vi "Test Bus of Buses.vi"() -> ()   [LabVIEW 2021]
uses:
  Source/Omni-Bus/Omni_Bus.lvclass
  Source/Omni-Bus/Support/Broad Types.ctl
  Source/Local Bus/Local Bus.lvclass
  <vilib>/Utility/Data Type/Type Definitions/Data Type.ctl
  <vilib>/Utility/Data Type/NI_Data Type.lvlib
  Source/Aggregator Bus/Aggregator Bus.lvclass
  C:/Users/Tim/Documents/GitHub/Omni-Bus/Source/Omni-Bus/Bus Access/Bus_Access.lvclass
  C:/Program Files (x86)/National Instruments/LabVIEW 2021/vi.lib/TSA/Abstract Data Classes/Abs_Types/Type/Abs_Type.lvclass
  C:/Users/Tim/Documents/GitHub/Omni-Bus/Source/Local Bus/Local Bus.lvclass
  Source/Omni-Bus/Support/Read/Read Time.vi
  Source/Omni-Bus/Support/Read/Read String.vi
  Source/Omni-Bus/Support/Read/Read Boolean.vi
  Source/Omni-Bus/Support/Write/Write String.vi
  Source/Omni-Bus/Support/Write/Write Boolean.vi
  <vilib>/TSA/Abstract Data Classes/Abs_Types/Time/Abs_Time.lvclass
  C:/Program Files (x86)/National Instruments/LabVIEW 2021/vi.lib/TSA/Abstract Data Classes/Abs_Types/Numeric/Abs_Numeric.lvclass
  C:/Program Files (x86)/National Instruments/LabVIEW 2021/vi.lib/TSA/Abstract Data Classes/Abs_Types/Value/Abs_Value.lvclass
  C:/Program Files (x86)/National Instruments/LabVIEW 2021/vi.lib/TSA/Abstract Data Classes/Abs_Types/Time/Abs_Time.lvclass
  C:/Users/Tim/Documents/GitHub/Omni-Bus/Source/Omni-Bus/Omni_Bus.lvclass
  C:/Users/Tim/Documents/GitHub/Omni-Bus/Source/Aggregator Bus/Aggregator Bus.lvclass
panel:
  in  "A 3":bool
  in  "B 3":dbl
  in  "C 3":string
  out "A 2":bool
  out "B 2":dbl
  out "C 2":string
  out "Time Stamp":timestamp
  in  "C":string
  in  "B":dbl
  in  "A":bool
  out "C":string
  out "B":dbl
  out "A":bool
  out "error out 3":errorcluster
  out "error out 2":errorcluster
  in  "Numeric 2":dbl
  in  "Tag 2":string
  in  "stop":bool
  out "Numeric":dbl
  in  "Tag":string
  out "error out":errorcluster
  out "Tags":string[](array[string])
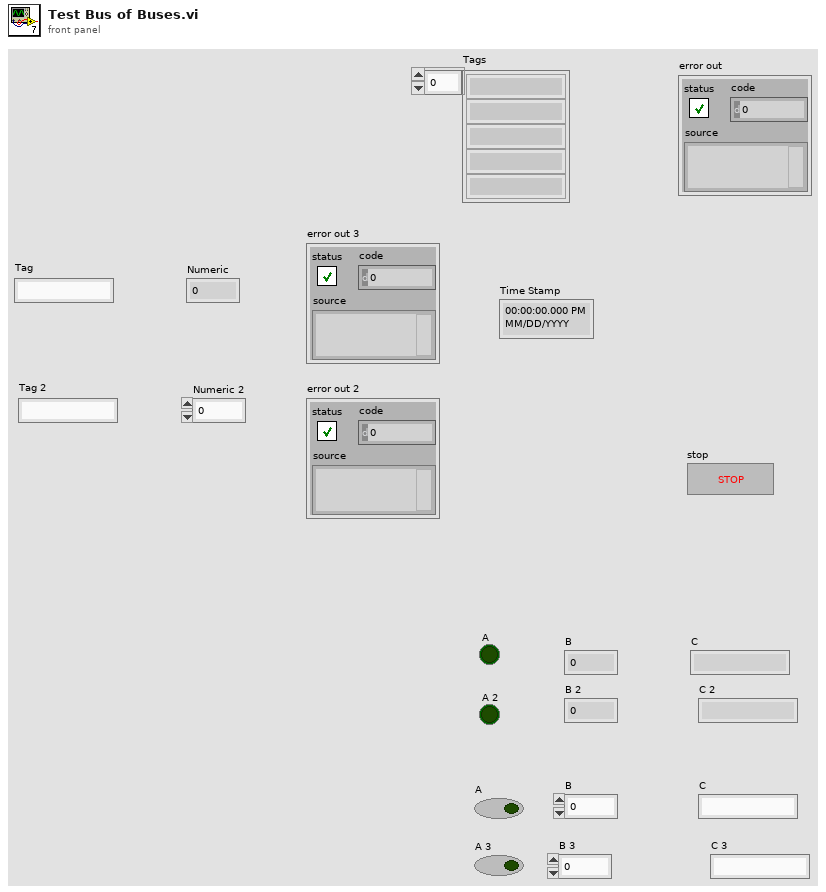
[diagram p1: front panel]
types:
  T1 = typedef "NI_Data Type.lvlib/Data Type.ctl" = enum8{"Invalid Type", "Void", "I8", "I16", "I32", "I64", "U8", "U16", "U32", "U64", "Single Float", "Double Float", "Extended Float", "Single Complex", "Double Complex", "Extended Complex", "Enum U8", "Enum U16", "Enum U32", "Enum U64", "Single Float With Unit", "Double Float With Unit", "Extended Float With Unit", "Single Complex with Unit", "Double Complex with Unit", "Extended Complex with Unit", "Boolean", "String", "Path", "Picture", "Tag", "Array", "Cluster", "Variant", "LV Variant", "Waveform", "Timestamp", "Digital Waveform", "Digital Data", "ExpressData", "Refnum", "External Data", "VI", "Poly VI", "LabVIEW Class Instance", "Fixed Point", "Set Collection", "Map Collection"}
  T2 = typedef "Omni_Bus.lvclass/Broad Types.ctl" = enum16{"All Tags", "NI Specific Type", "Boolean", "String", "Numeric", "Float", "Integer", "Collection", "All Value Types", "Non Value Types"}
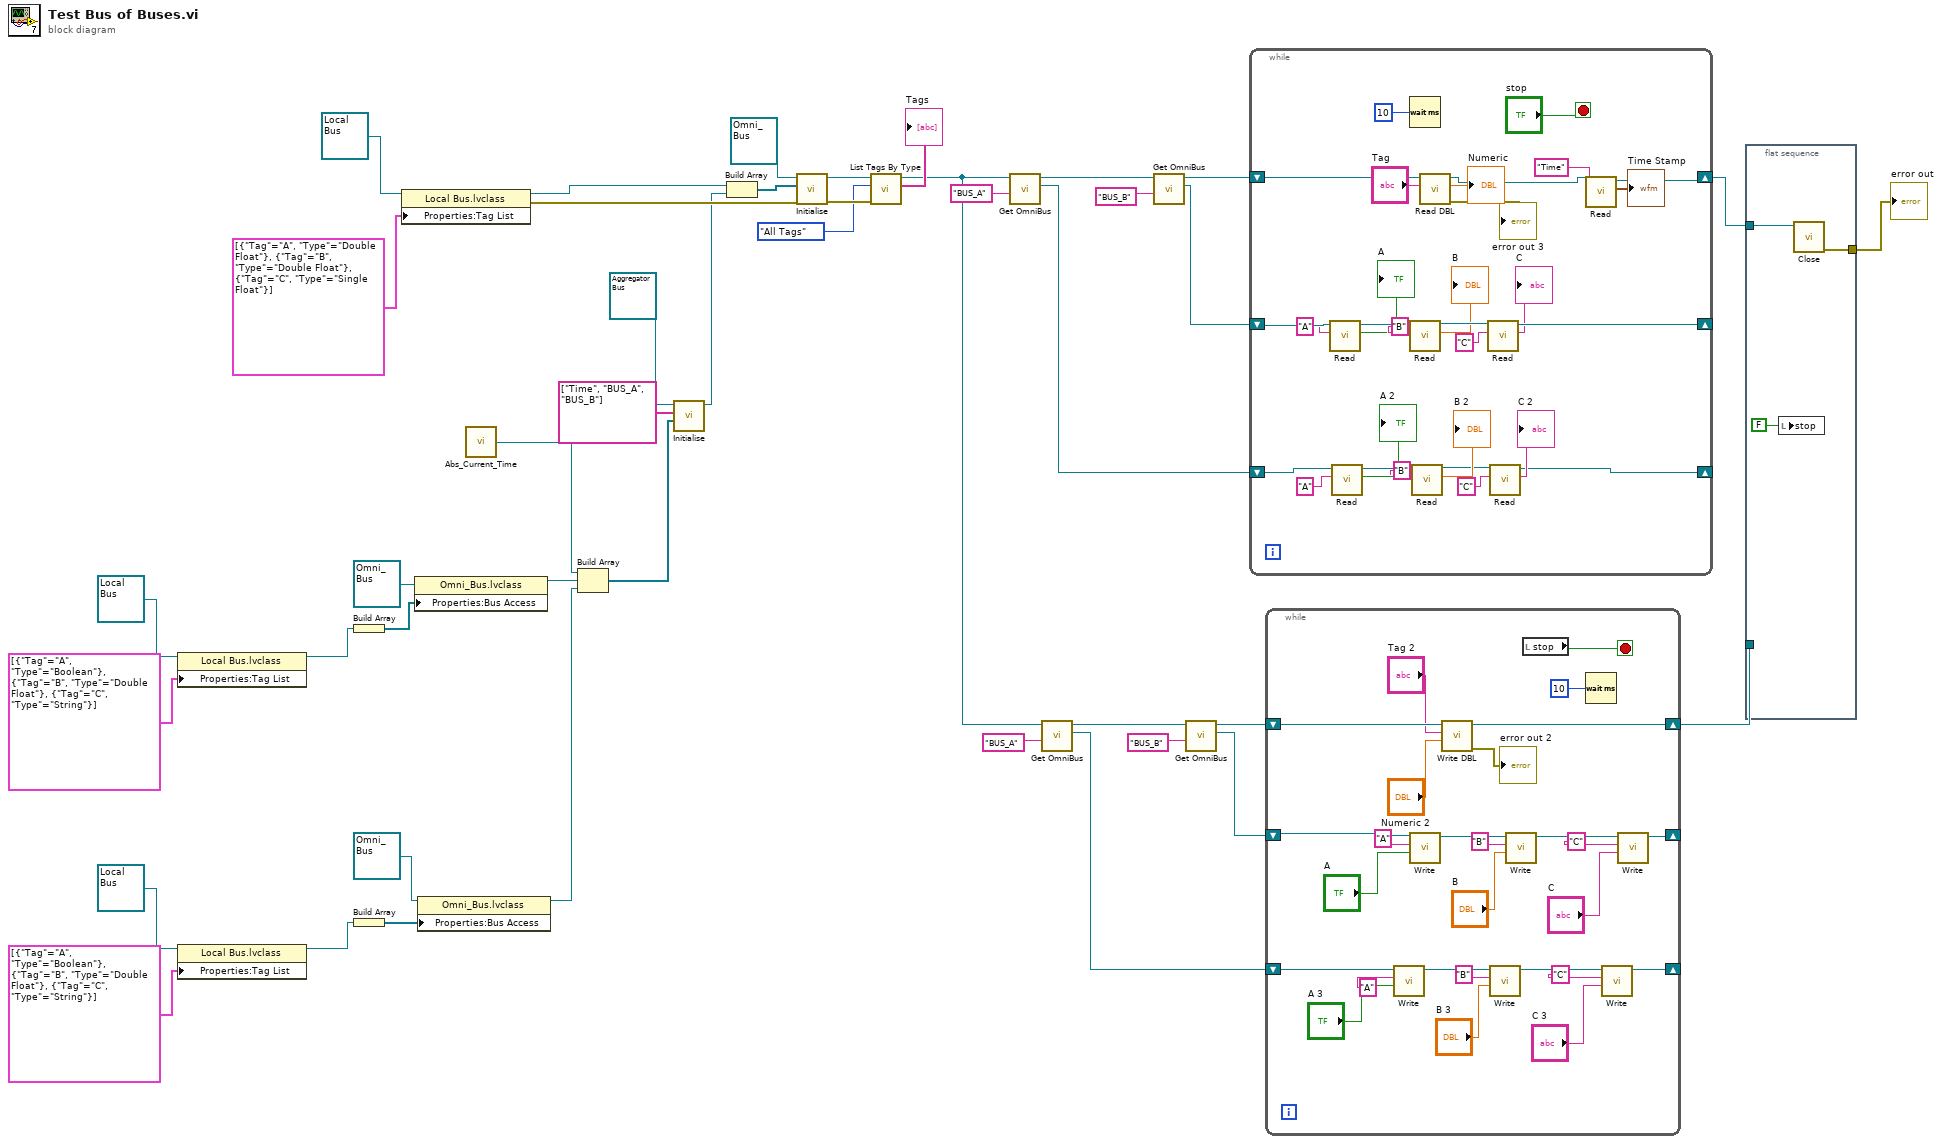
[diagram p0: block diagram]
diagram:
  n1 = property class="Local Bus.lvclass"(reference=refnum<class "Local Bus.lvclass"> refnum ("Local Bus.lvclass"), "Properties:Tag List"=cluster{"Tag":string, "Type":T1}[] [{"Tag"="A", "Type"=enum."Boolean"}, {"Tag"="B", "Type"=enum."Double Float"}, {"Tag"="C", "Type"=enum."String"}] ("Tag List")) -> (reference out=w24:refnum<class "Local Bus.lvclass">)  [unwired: 1 in, 1 out]
  n2 = property class="Local Bus.lvclass"(reference=refnum<class "Local Bus.lvclass"> refnum ("Local Bus.lvclass"), "Properties:Tag List"=cluster{"Tag":string, "Type":T1}[] [{"Tag"="A", "Type"=enum."Boolean"}, {"Tag"="B", "Type"=enum."Double Float"}, {"Tag"="C", "Type"=enum."String"}] ("Tag List")) -> (reference out=w23:refnum<class "Local Bus.lvclass">)  [unwired: 1 in, 1 out]
  n3 = Build Array(w24) -> (w18:refnum<class "Local Bus.lvclass">[])
  n4 = Build Array(w23) -> (w16:refnum<class "Local Bus.lvclass">[])
  n5 = property class="Local Bus.lvclass"(reference=refnum<class "Local Bus.lvclass"> refnum ("Local Bus.lvclass"), "Properties:Tag List"=cluster{"Tag":string, "Type":T1}[] [{"Tag"="A", "Type"=enum."Double Float"}, {"Tag"="B", "Type"=enum."Double Float"}, {"Tag"="C", "Type"=enum."Single Float"}] ("Tag List")) -> (reference out=w36:refnum<class "Local Bus.lvclass">, error out=w35:errorcluster)  [unwired: 1 in]
  n6 = property class="Omni_Bus.lvclass"(reference=refnum<class "Omni_Bus.lvclass"> refnum ("Var Bus in"), "Properties:Bus Access"=w18) -> (reference out=w19:refnum<class "Omni_Bus.lvclass">)  [unwired: 1 in, 1 out]
  n7 = property class="Omni_Bus.lvclass"(reference=refnum<class "Omni_Bus.lvclass"> refnum ("Var Bus in"), "Properties:Bus Access"=w16) -> (reference out=w15:refnum<class "Omni_Bus.lvclass">)  [unwired: 1 in, 1 out]
  n8 = call <vilib>:"Abs_Current_Time.vi"() -> ("Abs_Time.lvclass"=w14:refnum<class "Abs_Time.lvclass">)  [unwired: 5 in]
  n9 = Build Array(w14, w19, w15) -> (w28:refnum<class "Abs_Type.lvclass">[])
  n10 = call "Initialise.vi"("Values"=w28, "Tags"=string[] ["Time", "BUS_A", "BUS_B"], "Aggregator Bus in"=refnum<class "Aggregator Bus.lvclass"> refnum) -> ("Aggregator Bus out"=w30:refnum<class "Aggregator Bus.lvclass">)  [unwired: 7 in, 1 out]
  n11 = Build Array(w36, w30) -> (w42:refnum<class "Bus_Access.lvclass">[])
  n12 = call-dynamic "Initialise.vi"("error in (no error)"=w35, "Bus Access"=w42, "Var Bus in"=refnum<class "Omni_Bus.lvclass"> refnum) -> ("error out"=w40:errorcluster, "Var Bus out"=w41:refnum<class "Omni_Bus.lvclass">)  [unwired: 7 in]
  n13 = call-dynamic "List Tags By Type.vi"("error in (no error)"=w40, "Broad Types"=Broad_Types."All Tags", "Var Bus in"=w41) -> ("Tags"=→"Tags":string[], "Var Bus out"=w1:refnum<class "Omni_Bus.lvclass">)  [unwired: 5 in, 2 out]
  n14 = call-dynamic "Get OmniBus.vi"("Tag"="BUS_A", "Var Bus in"=w1) -> ("Value Out"=w6:refnum<class "Omni_Bus.lvclass">, "Var Bus out"=w7:refnum<class "Omni_Bus.lvclass">)  [unwired: 7 in, 1 out]
  n15 = call-dynamic "Get OmniBus.vi"("Tag"="BUS_A", "Var Bus in"=w1) -> ("Value Out"=w2:refnum<class "Omni_Bus.lvclass">, "Var Bus out"=w3:refnum<class "Omni_Bus.lvclass">)  [unwired: 7 in, 1 out]
  n16 = call-dynamic "Get OmniBus.vi"("Tag"="BUS_B", "Var Bus in"=w7) -> ("Value Out"=w10:refnum<class "Omni_Bus.lvclass">, "Var Bus out"=w11:refnum<class "Omni_Bus.lvclass">)  [unwired: 7 in, 1 out]
  n17 = call-dynamic "Get OmniBus.vi"("Tag"="BUS_B", "Var Bus in"=w3) -> ("Value Out"=w12:refnum<class "Omni_Bus.lvclass">, "Var Bus out"=w13:refnum<class "Omni_Bus.lvclass">)  [unwired: 7 in, 1 out]
  n18 = while {
    shift-right: [w56] -> w32
    shift-left: w11 -> [w73]
    shift-right: [w61] -> _
    shift-left: w10 -> [w66]
    shift-right: [w44] -> _
    shift-left: w6 -> [w45]
    stop <- "stop" stop-if-true
    n19 = call-poly "Read.vi"("Tag"="A" ("Tag 6"), "Var Bus in"=w66) -> ("Boolean"=→"A":bool, "Var Bus out"=w63:refnum<class "Omni_Bus.lvclass">)  [unwired: 7 in, 1 out]
    n20 = call-poly "Read.vi"("Tag"="A" ("Tag 6"), "Var Bus in"=w45) -> ("Boolean"=→"A 2":bool, "Var Bus out"=w48:refnum<class "Omni_Bus.lvclass">)  [unwired: 7 in, 1 out]
    n21 = Wait (ms)(milliseconds to wait=u32 10) -> ()  [unwired: 1 out]
    n22 = call-poly "Read.vi"("Tag"="B" ("Tag 7"), "Var Bus in"=w63) -> ("Numeric"=→"B":dbl, "Var Bus out"=w60:refnum<class "Omni_Bus.lvclass">)  [unwired: 7 in, 1 out]
    n23 = call-poly "Read.vi"("Tag"="B" ("Tag 7"), "Var Bus in"=w48) -> ("Numeric"=→"B 2":dbl, "Var Bus out"=w50:refnum<class "Omni_Bus.lvclass">)  [unwired: 7 in, 1 out]
    n24 = call "Read DBL.vi"("Tag"="Tag", "Var Bus in"=w73) -> ("error out"=→"error out 3":errorcluster, "Numeric"=→"Numeric":dbl, "Var Bus out"=w67:refnum<class "Omni_Bus.lvclass">)  [unwired: 7 in]
    n25 = call-poly "Read.vi"("Tag"="C" ("Tag 8"), "Var Bus in"=w60) -> ("String"=→"C":string, "Var Bus out"=w61:refnum<class "Omni_Bus.lvclass">)  [unwired: 7 in, 1 out]
    n26 = call-poly "Read.vi"("Tag"="C" ("Tag 8"), "Var Bus in"=w50) -> ("String"=→"C 2":string, "Var Bus out"=w44:refnum<class "Omni_Bus.lvclass">)  [unwired: 7 in, 1 out]
    n27 = call-poly "Read.vi"("Tag"="Time", "Var Bus in"=w67) -> ("Time Stamp"=→"Time Stamp":timestamp, "Var Bus out"=w56:refnum<class "Omni_Bus.lvclass">)  [unwired: 7 in, 1 out]
  }
  n28 = while {
    shift-right: [w94] -> w31
    shift-left: w13 -> [w100]
    shift-right: [w92] -> _
    shift-left: w12 -> [w93]
    shift-right: [w74] -> _
    shift-left: w2 -> [w75]
    stop <- w97 stop-if-true
    n29 = call-poly "Write.vi"("Boolean"="A 3", "Tag"="A" ("Tag 3"), "Omni_Bus in"=w75) -> ("Omni_Bus out"=w76:refnum<class "Omni_Bus.lvclass">)  [unwired: 7 in, 1 out]
    n30 = call-poly "Write.vi"("Boolean"="A", "Tag"="A" ("Tag 3"), "Omni_Bus in"=w93) -> ("Omni_Bus out"=w91:refnum<class "Omni_Bus.lvclass">)  [unwired: 7 in, 1 out]
    n31 = call "Write DBL.vi"("Numeric"="Numeric 2", "Tag"="Tag 2", "Omni_Bus in"=w100) -> ("error out"=→"error out 2":errorcluster, "Omni_Bus out"=w94:refnum<class "Omni_Bus.lvclass">)  [unwired: 7 in]
    n32 = call-poly "Write.vi"("Numeric"="B 3", "Tag"="B" ("Tag 4"), "Omni_Bus in"=w76) -> ("Omni_Bus out"=w77:refnum<class "Omni_Bus.lvclass">)  [unwired: 7 in, 1 out]
    n33 = call-poly "Write.vi"("Numeric"="B", "Tag"="B" ("Tag 4"), "Omni_Bus in"=w91) -> ("Omni_Bus out"=w90:refnum<class "Omni_Bus.lvclass">)  [unwired: 7 in, 1 out]
    n34 = local read "stop"() -> (w97:bool)
    n35 = Wait (ms)(milliseconds to wait=u32 10) -> ()  [unwired: 1 out]
    n36 = call-poly "Write.vi"("String"="C 3", "Tag"="C" ("Tag 5"), "Omni_Bus in"=w77) -> ("Omni_Bus out"=w74:refnum<class "Omni_Bus.lvclass">)  [unwired: 7 in, 1 out]
    n37 = call-poly "Write.vi"("String"="C", "Tag"="C" ("Tag 5"), "Omni_Bus in"=w90) -> ("Omni_Bus out"=w92:refnum<class "Omni_Bus.lvclass">)  [unwired: 7 in, 1 out]
  }
  n38 = flat-sequence {
    tunnel: [w103] -> w37
    tunnel: w32 -> [w102]
    tunnel: w31 -> [_]
    frame #0 {
      n39 = local write "stop"(FALSE ("stop")) -> ()
      n40 = call-dynamic "Close.vi"("Data in"=w102) -> ("error out"=w103:errorcluster)  [unwired: 9 in, 1 out]
    }
  }
  "error out" <- w37
